vi "TestExec.Prompt for entering Comment.vi"(11 "Comment":string) -> (3 "Comment Out":string)   [LabVIEW 2018]
panel:
  in  "OK Button":bool
  # "Enter Comment:"
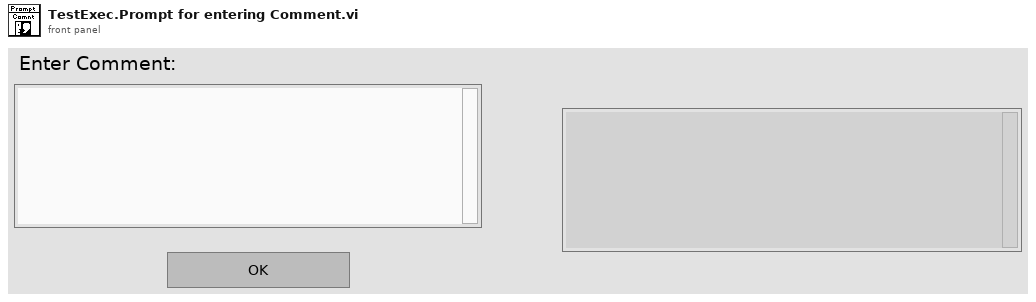
[diagram p1: front panel]
types:
  T1 = enum32{"Invalid", "Standard", "Closed", "Hidden", "Minimized", "Maximized"}
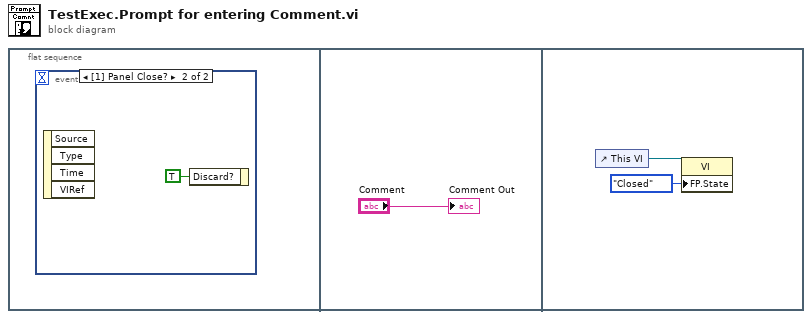
[diagram p0: block diagram]
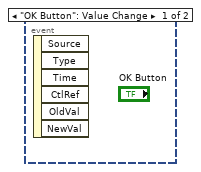
[diagram p2: hidden frame]
diagram:
  n1 = flat-sequence {
    frame #0 {
      n2 = event shown="[1] Panel Close?" {
        selector: _ -> [_ _]
        dyn-events: _ -> [_ _]
        timeout: _ -> [_ _]
        event "OK Button": Value Change {
          n3 = event-data() -> ()  [unwired: 1 in, 6 out]
        }
        event Panel Close? {
          n4 = event-data() -> ()  [unwired: 1 in, 4 out]
          n5 = event-data("Discard?"=TRUE) -> ()  [unwired: 1 in, 1 out]
        }
      }
    }
    frame #1 {
      "Comment Out" <- "Comment"
    }
    frame #2 {
      n6 = control-ref of="This VI"() -> (w4:refnum<vi>)
      n7 = property class="VI"(reference=w4, "FP.State"=T1."Closed" ("Front Panel Window:State")) -> ()  [unwired: 1 in, 2 out]
    }
  }
